vi "get_travel.vi"(0 "HGF_Agent.lvclass in":refnum<class "MoAgSy_AgentBase.lvclass">, 5 "error in (no error)":errorcluster) -> (11 "nextState?":enum16{"Ready", "stop", "travel"}(ring), 14 "HGF_Agent.lvclass out":refnum<class "MoAgSy_AgentBase.lvclass">, 19 "error out":errorcluster)   [LabVIEW 2009, in "MoAgSy_Base.lvlib" / "MoAgSy_AgentBase.lvclass"]
uses:
  MoAgSy_AgentBase.lvclass
  MoAgSy_AgentBase.lvclass/MoAgSy_AgentBase.ctl
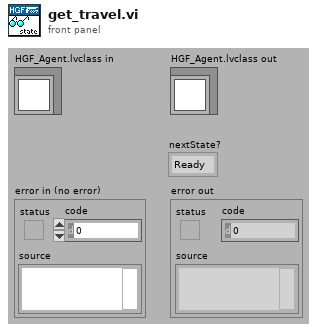
[diagram p1: front panel]
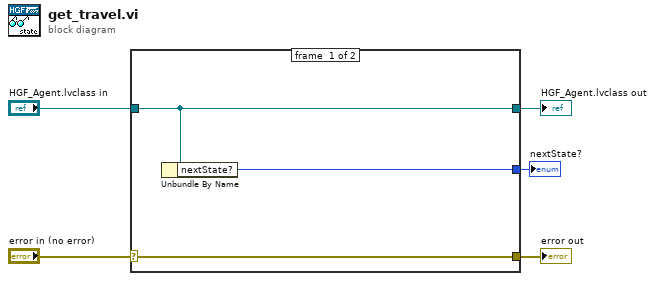
[diagram p0: block diagram]
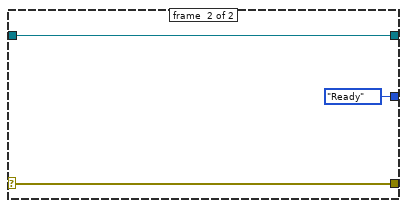
[diagram p2: hidden frame]
diagram:
  n1 = case shown="Error" "error in (no error)" {
    selector: "error in (no error)" -> [w8 w10]
    tunnel: [w8 w10] -> w4
    tunnel: [w7 w11] -> w2
    tunnel: "HGF_Agent.lvclass in" -> [w7 w11]
    tunnel: [w6 enum16{"Ready", "stop", "travel"}."Ready" ("nextState?")] -> w1
    frame #0 {
      n2 = Unbundle By Name(w7) -> ("nextState?"=w6:enum16{"Ready", "stop", "travel"})
    }
    frame #1 {
    }
  }
  "error out" <- w4
  "HGF_Agent.lvclass out" <- w2
  "nextState?" <- w1
